vi "Defer panel updates.vi"(9 "Defer Panel Updates":bool, 11 "Panel in":refnum<vi>) -> (3 "Panel out":refnum<vi>)   [LabVIEW 2017]
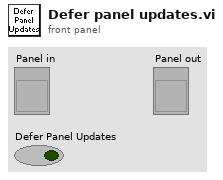
[diagram p1: front panel]
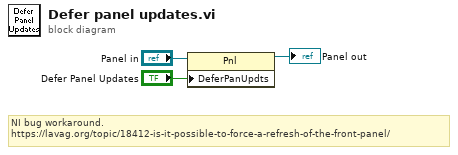
[diagram p0: block diagram]
diagram:
  # "NI bug workaround.\nhttps://lavag.org/topic/18412-is-it-possible-to-force-a-refresh-of-the-front-panel/"
  n1 = property on="Property Node" class="Pnl"(reference="Panel in", "DeferPanUpdts"="Defer Panel Updates") -> (reference out=→"Panel out":refnum<vi>)  [unwired: 1 in, 1 out]
